vi "MakeServerErrorCluster.vi"(4 "File Empty?":bool, 6 "Error Cluster in":T4, 8 "TabControl in":refnum<vi>, 9 "Number Cluster in":T5, 10 "# of Errors":i32, 11 "Log":T2={"Sent"="", "Reply"="", "MethodName"="", "success"=FALSE, "XML Direction 1"="", "XML Direction 2"="", "VI Name"="", "close reference"={"status"=FALSE, "code"=0, "source"=""}, "release queue"={"status"=FALSE, "code"=0, "source"=""}, "release notification"={"status"=FALSE, "code"=0, "source"=""}, "varaiant to data"={"status"=FALSE, "code"=0, "source"=""}, "console error"={"status"=FALSE, "code"=0, "source"=""}, "Time Stamp"="", "ROS"={"topic port"=0, "Node"="", "topic"="", "type"="", "node port"=0, "error "={"status"=FALSE, "code"=0, "source"=""}, "Direction"=enum."Node", "Update (ms)"=1, "write queue"=1}}) -> (1 "Server Errors":T3(array[cluster]), 2 "Error Cluster out":T4, 3 "Number Cluster out":T5)   [LabVIEW 2012]
uses:
  <userlib>/ROSforLV/ROS/Code/SubVIs/_ROSDirection.ctl
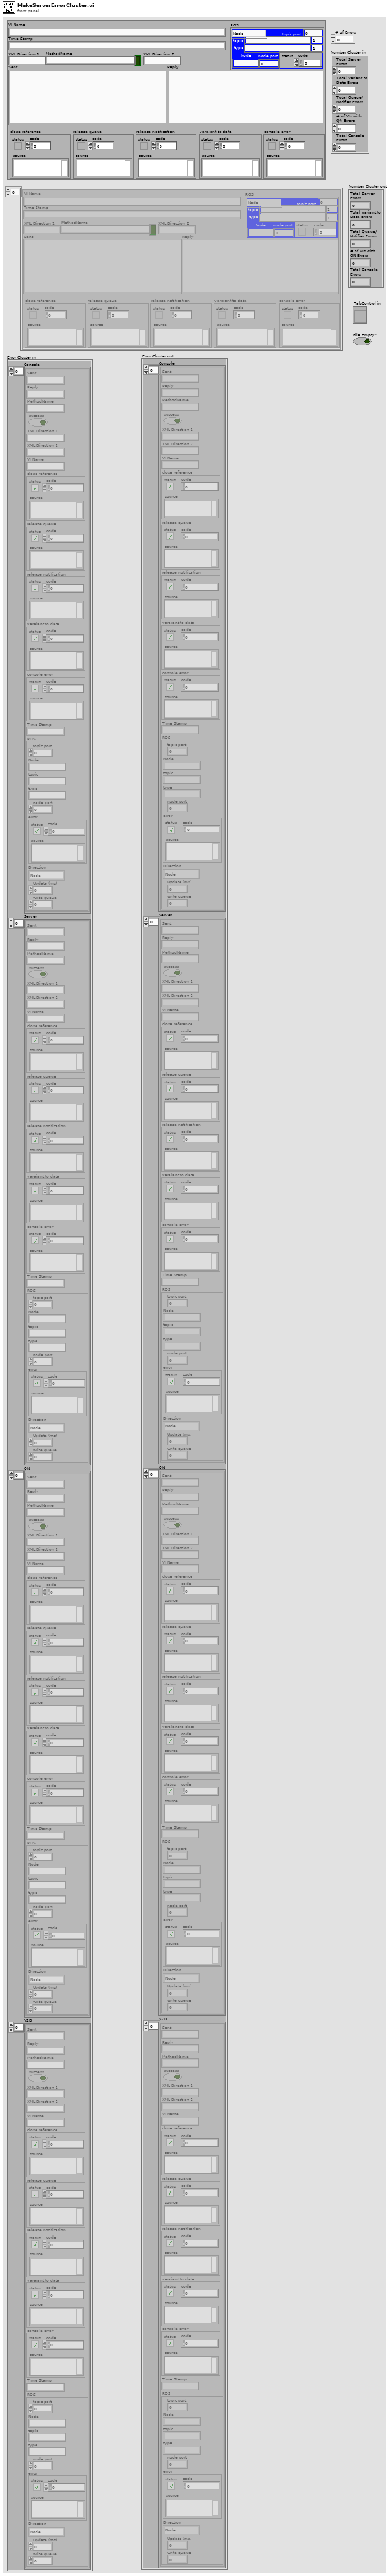
[diagram p1: front panel]
types:
  T1 = typedef "_ROSDirection.ctl" = enum16{"Node", "Publisher", "Subscriber", "Service Client"}
  T2 = cluster{"Sent":string, "Reply":string, "MethodName":string, "success":bool, "XML Direction 1":string, "XML Direction 2":string, "VI Name":string, "close reference":errorcluster, "release queue":errorcluster, "release notification":errorcluster, "varaiant to data":errorcluster, "console error":errorcluster, "Time Stamp":string, "ROS":cluster{"topic port":u16, "Node":string, "topic":string, "type":string, "node port":u32, "error ":errorcluster, "Direction":T1, "Update (ms)":u16, "write queue":u16}}
  T3 = cluster{"Sent":string, "Reply":string, "MethodName":string, "success":bool, "XML Direction 1":string, "XML Direction 2":string, "VI Name":string, "close reference":errorcluster, "release queue":errorcluster, "release notification":errorcluster, "varaiant to data":errorcluster, "console error":errorcluster, "Time Stamp":string, "ROS":cluster{"topic port":u16, "Node":string, "topic":string, "type":string, "node port":u32, "error ":errorcluster, "Direction":T1, "Update (ms)":u16, "write queue":u16}}[]
  T4 = cluster{"Console":cluster{"Sent":string, "Reply":string, "MethodName":string, "success":bool, "XML Direction 1":string, "XML Direction 2":string, "VI Name":string, "close reference":errorcluster, "release queue":errorcluster, "release notification":errorcluster, "varaiant to data":errorcluster, "console error":errorcluster, "Time Stamp":string, "ROS":cluster{"topic port":u16, "Node":string, "topic":string, "type":string, "node port":u32, "error ":errorcluster, "Direction":T1, "Update (ms)":u16, "write queue":u16}}[], "Server":cluster{"Sent":string, "Reply":string, "MethodName":string, "success":bool, "XML Direction 1":string, "XML Direction 2":string, "VI Name":string, "close reference":errorcluster, "release queue":errorcluster, "release notification":errorcluster, "varaiant to data":errorcluster, "console error":errorcluster, "Time Stamp":string, "ROS":cluster{"topic port":u16, "Node":string, "topic":string, "type":string, "node port":u32, "error ":errorcluster, "Direction":T1, "Update (ms)":u16, "write queue":u16}}[], "QN":cluster{"Sent":string, "Reply":string, "MethodName":string, "success":bool, "XML Direction 1":string, "XML Direction 2":string, "VI Name":string, "close reference":errorcluster, "release queue":errorcluster, "release notification":errorcluster, "varaiant to data":errorcluster, "console error":errorcluster, "Time Stamp":string, "ROS":cluster{"topic port":u16, "Node":string, "topic":string, "type":string, "node port":u32, "error ":errorcluster, "Direction":T1, "Update (ms)":u16, "write queue":u16}}[], "V2D":cluster{"Sent":string, "Reply":string, "MethodName":string, "success":bool, "XML Direction 1":string, "XML Direction 2":string, "VI Name":string, "close reference":errorcluster, "release queue":errorcluster, "release notification":errorcluster, "varaiant to data":errorcluster, "console error":errorcluster, "Time Stamp":string, "ROS":cluster{"topic port":u16, "Node":string, "topic":string, "type":string, "node port":u32, "error ":errorcluster, "Direction":T1, "Update (ms)":u16, "write queue":u16}}[]}
  T5 = cluster{"Total Server\nErrors":i32, "Total Variant to\nData Errors":i32, "Total Queue/\nNotifier Errors":i32, "# of VIs with\nQN Errors":i32, "Total Console\nErrors":i32}
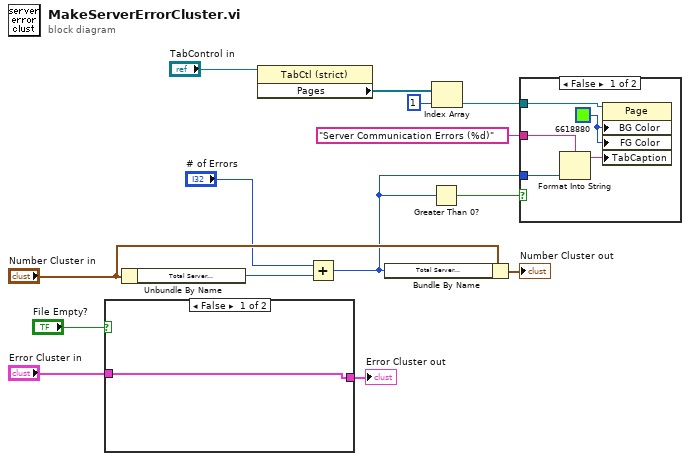
[diagram p0: block diagram]
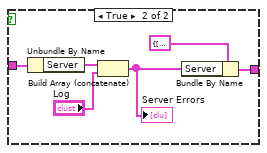
[diagram p2: hidden frame]
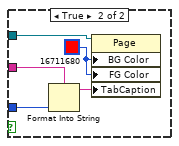
[diagram p3: hidden frame]
diagram:
  n1 = case shown="False" "File Empty?" {
    tunnel: [w15 w20] -> w11
    tunnel: "Error Cluster in" -> [w15 w19]
    frame False {
    }
    frame True {
      n2 = Unbundle By Name(w19) -> ("Server"=w18:T3)
      n3 = Build Array (concatenate)(w18, "Log") -> (w17:T3)
      "Server Errors" <- w17
      n4 = Bundle By Name(cluster=T4 {"Console"=[], "Server"=[], "QN"=[], "V2D"=[]}, "Server"=w17) -> (w20:T4)
    }
  }
  "Error Cluster out" <- w11
  n5 = Unbundle By Name("Number Cluster in") -> ("Total Server\nErrors"=w14:i32)
  n6 = property on="Property Node" class="TabCtl (strict)"(reference="TabControl in") -> ("Pages"=w7:refnum<vi>[])  [unwired: 1 in, 2 out]
  n7 = Add(x="# of Errors", y=w14) -> (x+y=w2:i32)
  n8 = Bundle By Name(cluster="Number Cluster in", "Total Server\nErrors"=w2) -> (→"Number Cluster out":T5)
  n9 = Greater Than 0?(x=w2) -> (x > 0?=w9:bool)
  n10 = Index Array(array=w7, index=1) -> (element=w6:refnum<vi>)
  n11 = case shown="False" w9 {
    tunnel: w6 -> [w24 w31]
    tunnel: w2 -> [w23 w28]
    tunnel: "Server Communication Errors (%d)" ("format string") -> [w22 w27]
    frame False {
      w26 = u32 6618880
      n12 = Format Into String(format string=w22, w23) -> (resulting string=w25:string)  [unwired: 2 in, 1 out]
      n13 = property on="Property Node" class="Page"(reference=w24, "BG Color"=w26, "FG Color"=w26, "TabCaption"=w25) -> ()  [unwired: 1 in, 2 out]
    }
    frame True {
      w30 = u32 16711680
      n14 = Format Into String(format string=w27, w28) -> (resulting string=w29:string)  [unwired: 2 in, 1 out]
      n15 = property on="Property Node" class="Page"(reference=w31, "BG Color"=w30, "FG Color"=w30, "TabCaption"=w29) -> ()  [unwired: 1 in, 2 out]
    }
  }
